vi "LVClass_WavefrontCorrectorSet Get Default WavefrontCorrectorParametersSetup.vi"(0 "WavefrontCorrectorSet in":refnum<class "WavefrontCorrectorSet.lvclass">, 11 "error in (no error)":errorcluster) -> (4 "WavefrontCorrectorSet out":refnum<class "WavefrontCorrectorSet.lvclass">, 6 "ListOfGettableParameter":T1[](array[typedef]), 8 "ListOfGettableSettableParameter":T1[](array[typedef]), 10 "AllValueDisable":T1[](array[typedef]), 15 "error out":errorcluster)   [LabVIEW 2020, in "WavefrontCorrectorSet.lvclass"]
uses:
  WavefrontCorrectorSet.lvclass
  Controls/CameraParametersSetup.ctl
  Controls/CameraParameters_Type.ctl
  Controls/ParameterID.ctl
  Controls/CameraParameters_Authorization.ctl
  Controls/CameraParameters_OnFlyAuthorization.ctl
  WavefrontCorrectorSet.lvclass/WavefrontCorrectorSet.ctl
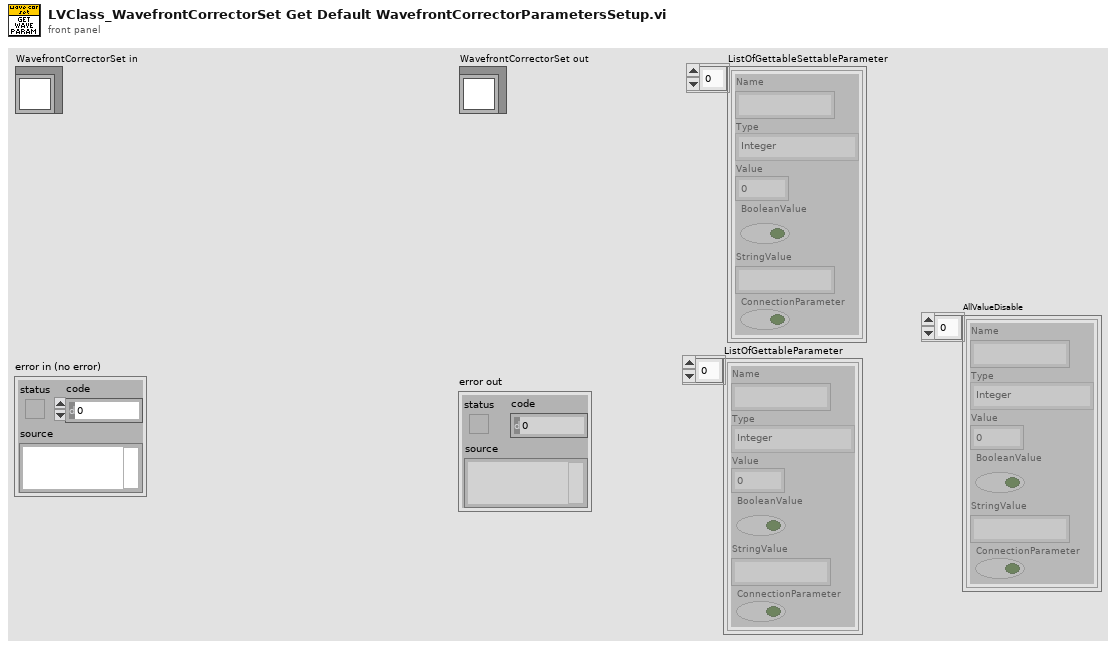
[diagram p1: front panel]
types:
  T1 = typedef "CameraParametersSetup.ctl" = cluster{"Name":string, "Type":T2, "Value":dbl, "BooleanValue":bool, "StringValue":string, "ConnectionParameter":bool}
  T2 = typedef "CameraParameters_Type.ctl" = enum16{"Integer", "Real", "String", "Boolean"}
  T3 = typedef "CameraParameters_Authorization.ctl" = enum16{"Disable", "Gettable", "Settable - Gettable"}
  T4 = typedef "CameraParameters_OnFlyAuthorization.ctl" = enum16{"None", "Gettable", "Settable", "Settable - Gettable"}
  T5 = typedef "ParameterID.ctl" = cluster{"Name":string, "ConnectionParameter?":bool, "Type":T2, "Authorization":T3, "OnFlyAuthorization":T4, "StringValue":string, "Value":dbl, "Min":dbl, "Max":dbl, "BooleanValue":bool, "StringParameterList":string[]}
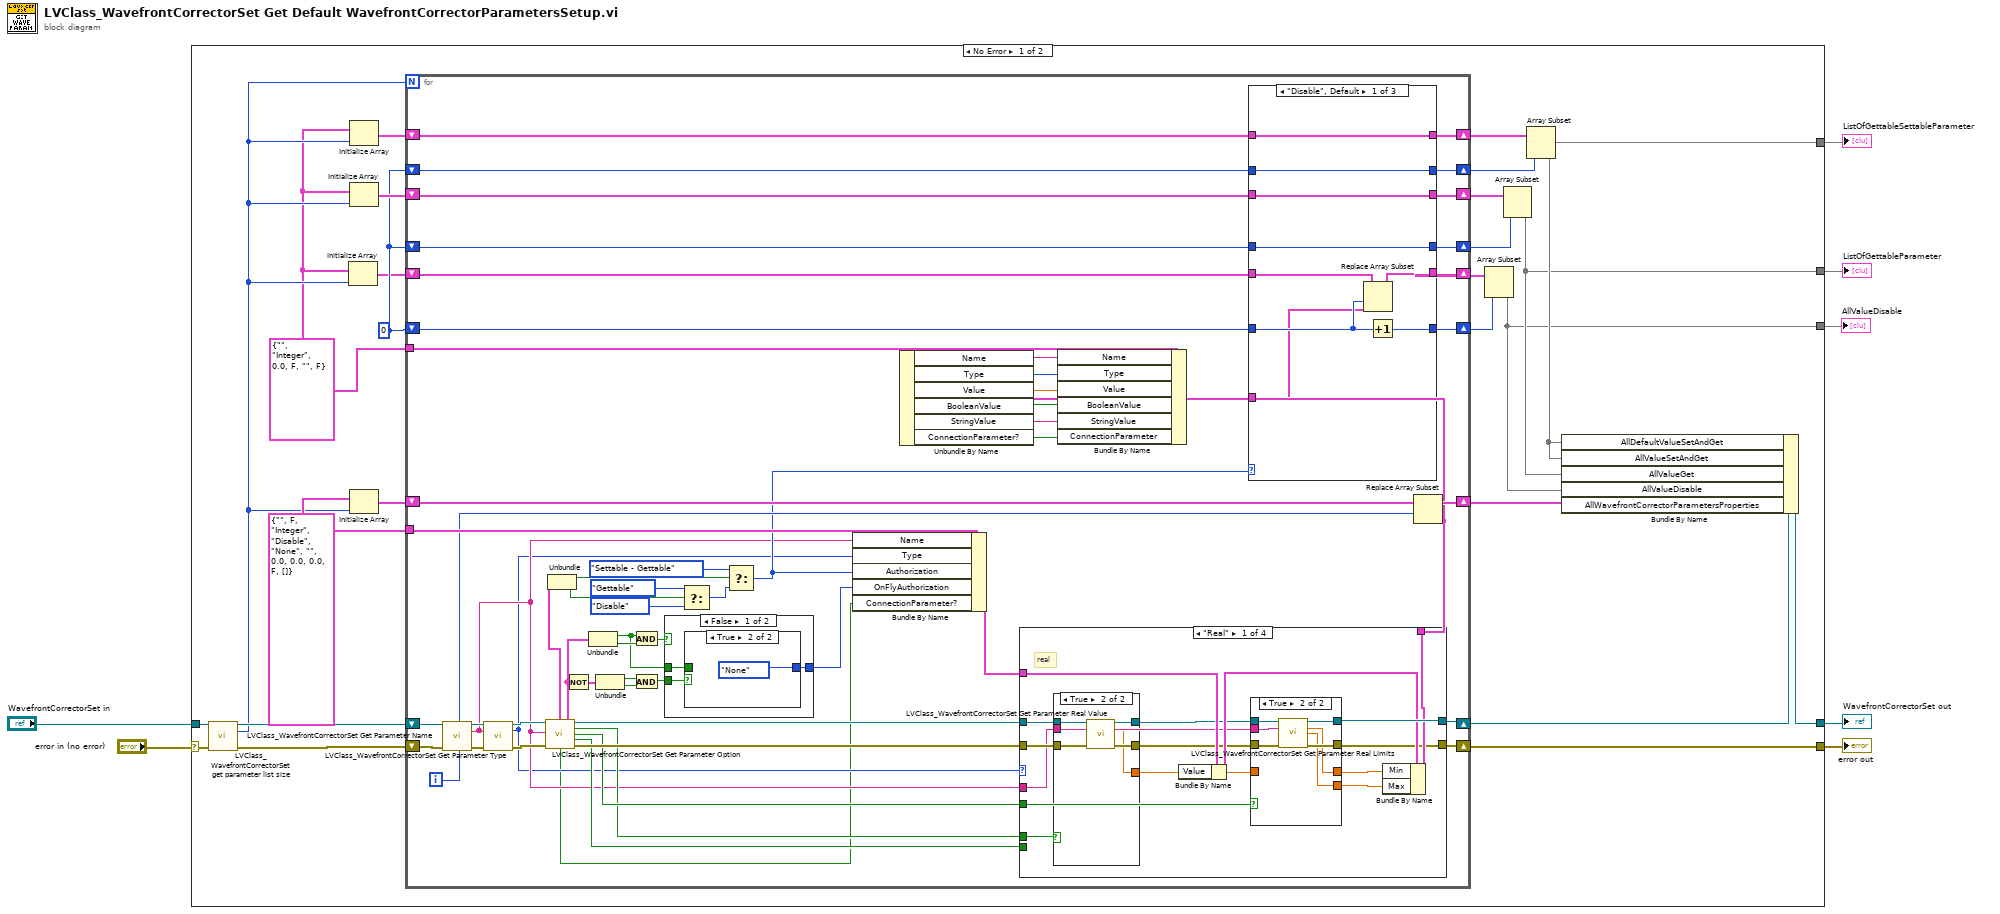
[diagram p0: block diagram]
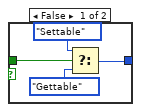
[diagram p2: hidden frame]
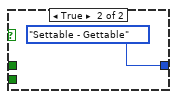
[diagram p3: hidden frame]
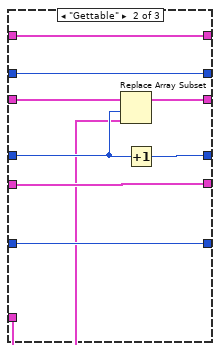
[diagram p4: hidden frame]
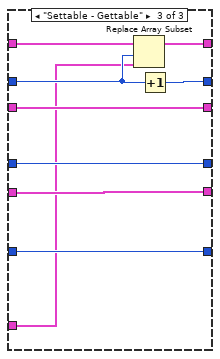
[diagram p5: hidden frame]
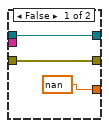
[diagram p6: hidden frame]
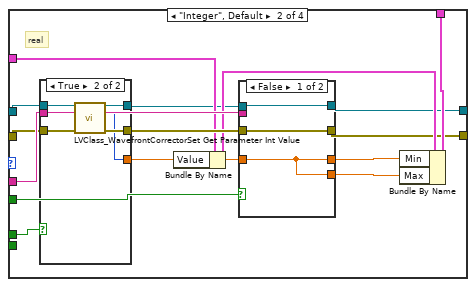
[diagram p8: hidden frame]
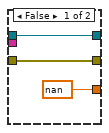
[diagram p9: hidden frame]
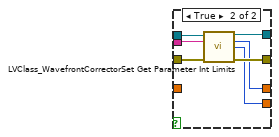
[diagram p10: hidden frame]
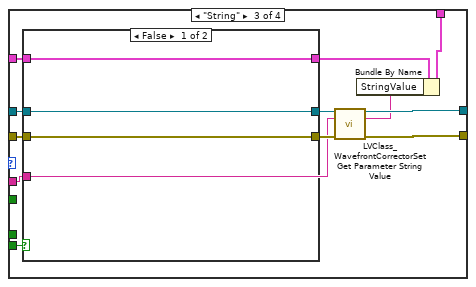
[diagram p11: hidden frame]
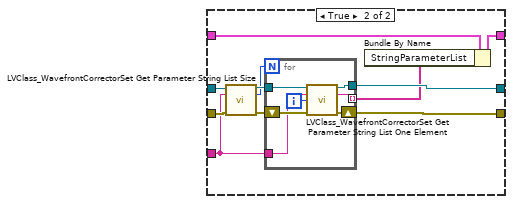
[diagram p12: hidden frame]
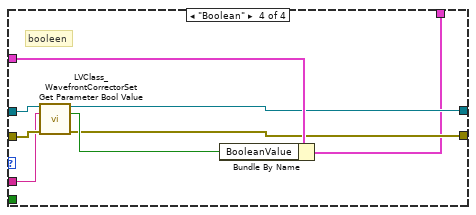
[diagram p13: hidden frame]
diagram:
  n1 = case shown="No Error" "error in (no error)" {
    selector: "error in (no error)" -> [w30 w238]
    tunnel: [w29 w238] -> w6
    tunnel: [w31 w237] -> w4
    tunnel: "WavefrontCorrectorSet in" -> [w28 w237]
    tunnel: [w10 _] -> w3
    tunnel: [w11 _] -> w2
    tunnel: [w9 _] -> w1
    frame No Error {
      w8 = T1 {"Name"="", "Type"=enum."Integer", "Value"=0.0, "BooleanValue"=FALSE, "StringValue"="", "ConnectionParameter"=FALSE} ("CameraParametersSetup")
      w16 = 0
      w24 = T5 {"Name"="", "ConnectionParameter?"=FALSE, "Type"=enum."Integer", "Authorization"=enum."Disable", "OnFlyAuthorization"=enum."None", "StringValue"="", "Value"=0.0, "Min"=0.0, "Max"=0.0, "BooleanValue"=FALSE, "StringParameterList"=[]} ("CameraParameters")
      n2 = call "LVClass_WavefrontCorrectorSet get parameter list size.vi"("WavefrontCorrectorSet in"=w28, "error in (no error)"=w30) -> ("WavefrontCorrectorSet out"=w27:refnum<class "WavefrontCorrectorSet.lvclass">, "ParametersListSize"=w14:i32, "error out"=w32:errorcluster)  [unwired: 11 in]
      n3 = Initialize Array(w8, w14) -> (w15:T1[])
      n4 = Initialize Array(w8, w14) -> (w19:T1[])
      n5 = Initialize Array(w8, w14) -> (w21:T1[])
      n6 = Initialize Array(w24, w14) -> (w25:T5[])
      n7 = for {
        N: w14 -> [_]
        tunnel: w24 -> [w87]
        shift-right: [w86] -> w29
        shift-left: w32 -> [w90]
        shift-right: [w85] -> w26
        shift-left: w27 -> [w91]
        shift-right: [w73] -> w23
        shift-left: w25 -> [w74]
        shift-right: [w70] -> w20
        shift-left: w16 -> [w71]
        shift-right: [w69] -> w22
        shift-left: w21 -> [w67]
        shift-right: [w65] -> w18
        shift-left: w19 -> [w66]
        shift-right: [w63] -> w17
        shift-left: w16 -> [w64]
        shift-right: [w48] -> w12
        shift-left: w16 -> [w47]
        shift-right: [w45] -> w13
        shift-left: w15 -> [w46]
        tunnel: w8 -> [w38]
        i -> [w72]
        n8 = call "LVClass_WavefrontCorrectorSet Get Parameter Name.vi"("WavefrontCorrectorSet in"=w91, "index"=w72, "error in (no error)"=w90) -> ("WavefrontCorrectorSet out"=w89:refnum<class "WavefrontCorrectorSet.lvclass">, "parameter_name"=w44:string, "error out"=w88:errorcluster)  [unwired: 10 in]
        n9 = call "LVClass_WavefrontCorrectorSet Get Parameter Type.vi"("WavefrontCorrectorSet in"=w89, "parameter_name"=w44, "error in (no error)"=w88) -> ("WavefrontCorrectorSet out"=w84:refnum<class "WavefrontCorrectorSet.lvclass">, "Type"=w43:T2, "error out"=w83:errorcluster)  [unwired: 10 in]
        n10 = call "LVClass_WavefrontCorrectorSet Get Parameter Option.vi"("WavefrontCorrectorSet in"=w84, "parameter_name"=w44, "error in (no error)"=w83) -> ("Settable-Gettable?"=w60:cluster{"Settable":bool, "Gettable":bool}, "WavefrontCorrectorSet out"=w82:refnum<class "WavefrontCorrectorSet.lvclass">, "DefaultValueExist"=w62:bool, "minmax"=w75:bool, "String enum"=w61:bool, "is_connection_parameter?"=w33:bool, "Settable-Gettable on fly?"=w53:cluster{"Settable":bool, "Gettable":bool}, "error out"=w81:errorcluster)  [unwired: 5 in]
        n11 = Unbundle(w60) -> ("Settable"=w59:bool, "Gettable"=w58:bool)
        n12 = Not(x=w53) -> (.not. x?=w51:cluster{"Settable":bool, "Gettable":bool})
        n13 = Unbundle(w53) -> ("Settable"=w50:bool, "Gettable"=w57:bool)
        n14 = Unbundle(w51) -> ("Settable"=w52:bool, "Gettable"=w55:bool)
        n15 = And(x=w50, y=w57) -> (x .and. y?=w56:bool)
        n16 = And(x=w52, y=w55) -> (x .and. y?=w54:bool)
        n17 = case shown="False" w56 {
          tunnel: [w93 CameraParameters_OnFlyAuthorization."Settable - Gettable" ("OnFlyAuthorization")] -> w49
          tunnel: w54 -> [w94 _]
          tunnel: w50 -> [w92 _]
          frame False {
            n18 = case shown="True" w94 {
              tunnel: [w98 CameraParameters_OnFlyAuthorization."None" ("OnFlyAuthorization")] -> w93
              tunnel: w92 -> [w95 _]
              frame False {
                n19 = Select(t=CameraParameters_OnFlyAuthorization."Settable" ("OnFlyAuthorization"), s=w95, f=CameraParameters_OnFlyAuthorization."Gettable" ("OnFlyAuthorization")) -> (s? t:f=w98:T4)
              }
              frame True {
              }
            }
          }
          frame True {
          }
        }
        n20 = Select(t=CameraParameters_Authorization."Gettable" ("Authorization"), s=w58, f=CameraParameters_Authorization."Disable") -> (s? t:f=w78:T3)
        n21 = Select(t=CameraParameters_Authorization."Settable - Gettable", s=w59, f=w78) -> (s? t:f=w68:T3)
        n22 = Bundle By Name(cluster=w87, "Name"=w44, "Type"=w43, "Authorization"=w68, "OnFlyAuthorization"=w49, "ConnectionParameter?"=w33) -> (w76:T5)
        n23 = case shown="\"Real\"" w43 {
          tunnel: w76 -> [w136 w169 w199 w235]
          tunnel: w44 -> [w132 w173 w201 w232]
          tunnel: [w128 w165 w203 w230] -> w86
          tunnel: w82 -> [w138 w163 w207 w234]
          tunnel: w81 -> [w133 w171 w206 w233]
          tunnel: [w137 w166 w204 w231] -> w85
          tunnel: w62 -> [w139 w172 _ _]
          tunnel: w75 -> [w142 w176 _ _]
          tunnel: w61 -> [_ _ w197 _]
          tunnel: [w134 w167 w196 w229] -> w39
          frame "Real" {
            # "real"
            n24 = case shown="True" w139 {
              tunnel: w138 -> [w145 w151]
              tunnel: w133 -> [w144 w147]
              tunnel: [w144 w150] -> w130
              tunnel: [w145 w149] -> w131
              tunnel: [nan ("f") w148] -> w129
              tunnel: w132 -> [_ w146]
              frame False {
              }
              frame True {
                n25 = call "LVClass_WavefrontCorrectorSet Get Parameter Real Value.vi"("WavefrontCorrectorSet in"=w151, "parameter_name"=w146, "error in (no error)"=w147) -> ("WavefrontCorrectorSet out"=w149:refnum<class "WavefrontCorrectorSet.lvclass">, "Value"=w148:dbl, "error out"=w150:errorcluster)  [unwired: 10 in]
              }
            }
            n26 = Bundle By Name(cluster=w136, "Value"=w129) -> (w135:T5)
            n27 = case shown="True" w142 {
              tunnel: w132 -> [_ w161]
              tunnel: [w154 w160] -> w128
              tunnel: [w153 w159] -> w137
              tunnel: w130 -> [w154 w158]
              tunnel: [w152 w157] -> w141
              tunnel: [w152 w156] -> w140
              tunnel: w131 -> [w153 w155]
              tunnel: w129 -> [w152 _]
              frame False {
              }
              frame True {
                n28 = call "LVClass_WavefrontCorrectorSet Get Parameter Real Limits.vi"("WavefrontCorrectorSet in"=w155, "parameter_name"=w161, "error in (no error)"=w158) -> ("WavefrontCorrectorSet out"=w159:refnum<class "WavefrontCorrectorSet.lvclass">, "min"=w157:dbl, "max"=w156:dbl, "error out"=w160:errorcluster)  [unwired: 9 in]
              }
            }
            n29 = Bundle By Name(cluster=w135, "Min"=w141, "Max"=w140) -> (w134:T5)
          }
          frame "Integer", Default {
            # "real"
            n30 = case shown="True" w172 {
              tunnel: w173 -> [_ w185]
              tunnel: w163 -> [w179 w184]
              tunnel: w171 -> [w178 w183]
              tunnel: [w178 w182] -> w170
              tunnel: [w179 w181] -> w162
              tunnel: [nan ("f") w180] -> w164
              frame False {
              }
              frame True {
                n31 = call "LVClass_WavefrontCorrectorSet Get Parameter Int Value.vi"("WavefrontCorrectorSet in"=w184, "parameter_name"=w185, "error in (no error)"=w183) -> ("WavefrontCorrectorSet out"=w181:refnum<class "WavefrontCorrectorSet.lvclass">, "Value"=w180:i32, "error out"=w182:errorcluster)  [unwired: 10 in]
              }
            }
            n32 = Bundle By Name(cluster=w169, "Value"=w164) -> (w168:T5)
            n33 = case shown="False" w176 {
              tunnel: w173 -> [_ w195]
              tunnel: [w188 w194] -> w165
              tunnel: [w187 w193] -> w166
              tunnel: w162 -> [w187 w192]
              tunnel: w170 -> [w188 w191]
              tunnel: [w186 w190] -> w175
              tunnel: [w186 w189] -> w174
              tunnel: w164 -> [w186 _]
              frame False {
              }
              frame True {
                n34 = call "LVClass_WavefrontCorrectorSet Get Parameter Int Limits.vi"("WavefrontCorrectorSet in"=w192, "parameter_name"=w195, "error in (no error)"=w191) -> ("WavefrontCorrectorSet out"=w193:refnum<class "WavefrontCorrectorSet.lvclass">, "min"=w190:i32, "max"=w189:i32, "error out"=w194:errorcluster)  [unwired: 9 in]
              }
            }
            n35 = Bundle By Name(cluster=w168, "Min"=w175, "Max"=w174) -> (w167:T5)
          }
          frame "String" {
            n36 = case shown="False" w197 {
              tunnel: w207 -> [w210 w221]
              tunnel: w206 -> [w209 w220]
              tunnel: [w210 w216] -> w205
              tunnel: [w209 w215] -> w202
              tunnel: w201 -> [_ w211]
              tunnel: w199 -> [w208 w214]
              tunnel: [w208 w212] -> w198
              frame False {
              }
              frame True {
                n37 = call "LVClass_WavefrontCorrectorSet Get Parameter String List Size.vi"("WavefrontCorrectorSet in"=w221, "parameter name"=w211, "error in (no error)"=w220) -> ("WavefrontCorrectorSet out"=w219:refnum<class "WavefrontCorrectorSet.lvclass">, "size"=w217:i32, "error out"=w218:errorcluster)  [unwired: 10 in]
                n38 = for {
                  N: w217 -> [_]
                  tunnel: w211 -> [w226]
                  tunnel: [w223] -> w216
                  tunnel: w219 -> [w228]
                  shift-right: [w222] -> w215
                  shift-left: w218 -> [w227]
                  tunnel: [w224] -> w213 mode=indexing
                  i -> [w225]
                  n39 = call "LVClass_WavefrontCorrectorSet Get Parameter String List One Element.vi"("WavefrontCorrectorSet in"=w228, "parameter name"=w226, "index"=w225, "error in (no error)"=w227) -> ("WavefrontCorrectorSet out"=w223:refnum<class "WavefrontCorrectorSet.lvclass">, "value"=w224:string, "error out"=w222:errorcluster)  [unwired: 9 in]
                }
                n40 = Bundle By Name(cluster=w214, "StringParameterList"=w213) -> (w212:T5)
              }
            }
            n41 = call "LVClass_WavefrontCorrectorSet Get Parameter String Value.vi"("WavefrontCorrectorSet in"=w205, "parameter name"=w201, "error in (no error)"=w202) -> ("WavefrontCorrectorSet out"=w204:refnum<class "WavefrontCorrectorSet.lvclass">, "Value"=w200:string, "error out"=w203:errorcluster)  [unwired: 10 in]
            n42 = Bundle By Name(cluster=w198, "StringValue"=w200) -> (w196:T5)
          }
          frame "Boolean" {
            # "booleen"
            n43 = call "LVClass_WavefrontCorrectorSet Get Parameter Bool Value.vi"("WavefrontCorrectorSet in"=w234, "parameter_name"=w232, "error in (no error)"=w233) -> ("WavefrontCorrectorSet out"=w231:refnum<class "WavefrontCorrectorSet.lvclass">, "Value"=w236:bool, "error out"=w230:errorcluster)  [unwired: 10 in]
            n44 = Bundle By Name(cluster=w235, "BooleanValue"=w236) -> (w229:T5)
          }
        }
        n45 = Unbundle By Name(w39) -> ("Name"=w34:string, "Type"=w40:T2, "Value"=w41:dbl, "BooleanValue"=w42:bool, "StringValue"=w37:string, "ConnectionParameter?"=w36:bool)
        n46 = Bundle By Name(cluster=w38, "Name"=w34, "Type"=w40, "Value"=w41, "BooleanValue"=w42, "StringValue"=w37, "ConnectionParameter"=w36) -> (w35:T1)
        n47 = case shown="\"Disable\", Default" w68 {
          tunnel: w71 -> [w108 w118 w122]
          tunnel: [w108 w117 w122] -> w70
          tunnel: [w109 w116 w123] -> w69
          tunnel: w67 -> [w109 w115 w123]
          tunnel: w66 -> [w103 w113 w127]
          tunnel: [w103 w113 w126] -> w65
          tunnel: w64 -> [w102 w114 w125]
          tunnel: [w102 w114 w124] -> w63
          tunnel: [w104 w111 w120] -> w48
          tunnel: w47 -> [w105 w111 w120]
          tunnel: w46 -> [w107 w112 w121]
          tunnel: [w106 w112 w121] -> w45
          tunnel: w35 -> [w101 w110 w119]
          frame "Disable", Default {
            n48 = Replace Array Subset(array=w107, new element=w101, index=w105) -> (w106:T1[])
            n49 = Increment(x=w105) -> (x+1=w104:i32)
          }
          frame "Gettable" {
            n50 = Replace Array Subset(array=w115, new element=w110, index=w118) -> (w116:T1[])
            n51 = Increment(x=w118) -> (x+1=w117:i32)
          }
          frame "Settable - Gettable" {
            n52 = Replace Array Subset(array=w127, new element=w119, index=w125) -> (w126:T1[])
            n53 = Increment(x=w125) -> (x+1=w124:i32)
          }
        }
        n54 = Replace Array Subset(array=w74, new element=w39, index=w72) -> (w73:T5[])
      }
      n55 = Array Subset(array=w13, length=w12) -> (w9:T1[])  [unwired: 1 in]
      n56 = Array Subset(array=w22, length=w20) -> (w10:T1[])  [unwired: 1 in]
      n57 = Array Subset(array=w18, length=w17) -> (w11:T1[])  [unwired: 1 in]
      n58 = Bundle By Name(cluster=w26, "AllDefaultValueSetAndGet"=w11, "AllValueSetAndGet"=w11, "AllValueGet"=w10, "AllValueDisable"=w9, "AllWavefrontCorrectorParametersProperties"=w23) -> (w31:refnum<class "WavefrontCorrectorSet.lvclass">)
    }
    frame Error {
    }
  }
  "error out" <- w6
  "WavefrontCorrectorSet out" <- w4
  "ListOfGettableParameter" <- w3
  "ListOfGettableSettableParameter" <- w2
  "AllValueDisable" <- w1
